vi "PWM Output Write.vi"(8 "error in":errorcluster, 10 "PWM Output Write":cluster{"duty cycle":dbl, "frequency":dbl}[](array[cluster]), 11 "NI PWM Output in":refnum<class "NI PWM Output.lvclass">) -> (0 "error out":errorcluster, 3 "NI PWM Output out":refnum<class "NI PWM Output.lvclass">)   [LabVIEW 2023, in "HardwareAbstractionLayer_LVOOP.lvlib" / "NI PWM Output.lvclass"]
uses:
  NI PWM Output.lvclass
  NI PWM Output.lvclass/NI PWM Output.ctl
  <vilib>/DAQmx/write.llb/DAQmx Write (Counter 1D Frequency NChan 1Samp).vi
  <vilib>/DAQmx/miscellaneous.llb/DAQmx Fill In Error Info.vi
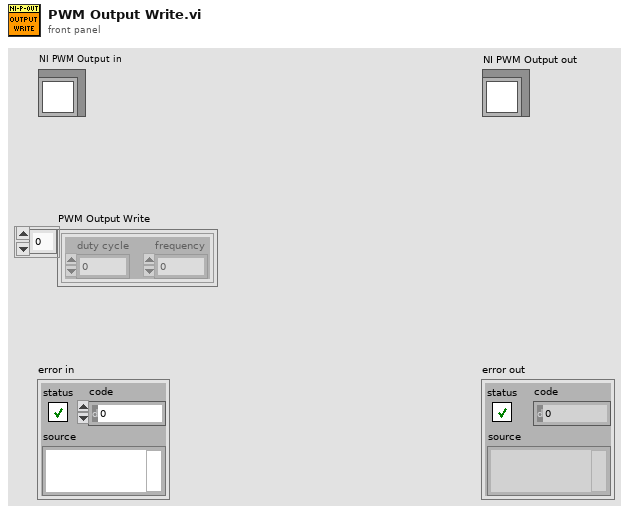
[diagram p1: front panel]
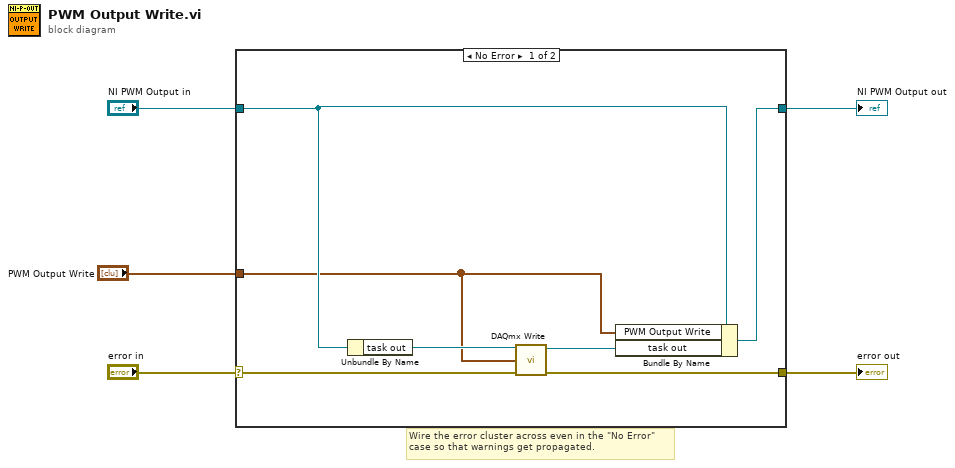
[diagram p0: block diagram]
diagram:
  # "Wire the error cluster across even in the \"No Error\"\ncase so that warnings get propagated."
  n1 = case shown="No Error" "error in" {
    selector: "error in" -> [w12 w14]
    tunnel: [w11 w14] -> w4
    tunnel: [w9 w13] -> w2
    tunnel: "NI PWM Output in" -> [w10 w13]
    tunnel: "PWM Output Write" -> [w6 _]
    frame No Error {
      n2 = Unbundle By Name(w10) -> ("task out"=w7:refnum<k21>)
      n3 = call-poly <vilib>:"DAQmx Write.vi"("task/channels in"=w7, "data"=w6, "error in"=w12) -> ("task out"=w8:refnum<k21>, "error out"=w11:errorcluster)  [unwired: 10 in, 1 out]
      n4 = Bundle By Name(cluster=w10, "PWM Output Write"=w6, "task out"=w8) -> (w9:refnum<class "NI PWM Output.lvclass">)
    }
    frame Error {
    }
  }
  "error out" <- w4
  "NI PWM Output out" <- w2
